vi "Global Current Values.vi"() -> ()   [LabVIEW 2016]
panel:
  out "Average Current":dbl
  out "Current Values":dbl[](array[numeric])
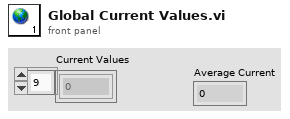
[diagram p1: front panel]
diagram:
